vi "SetFrameTime.vi"(3 "错误输入":errorcluster, 4 "IMAQdx Session In":T1, 5 "帧间隔/us":i64) -> (0 "错误输出":errorcluster, 1 "IMAQdx Session Out":T1, 2 "帧率/FPS":dbl)   [LabVIEW 2012]
uses:
  <vilib>/userDefined/High Color/IMAQdx.ctl
  <resource>/objmgr/imaqdx.rc
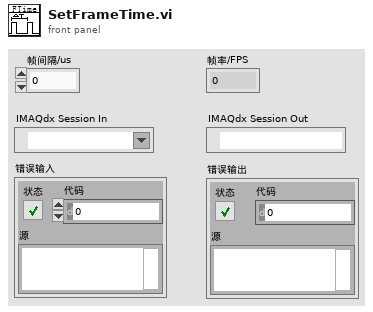
[diagram p1: front panel]
types:
  T1 = typedef "IMAQdx.ctl" = refnum<k21>
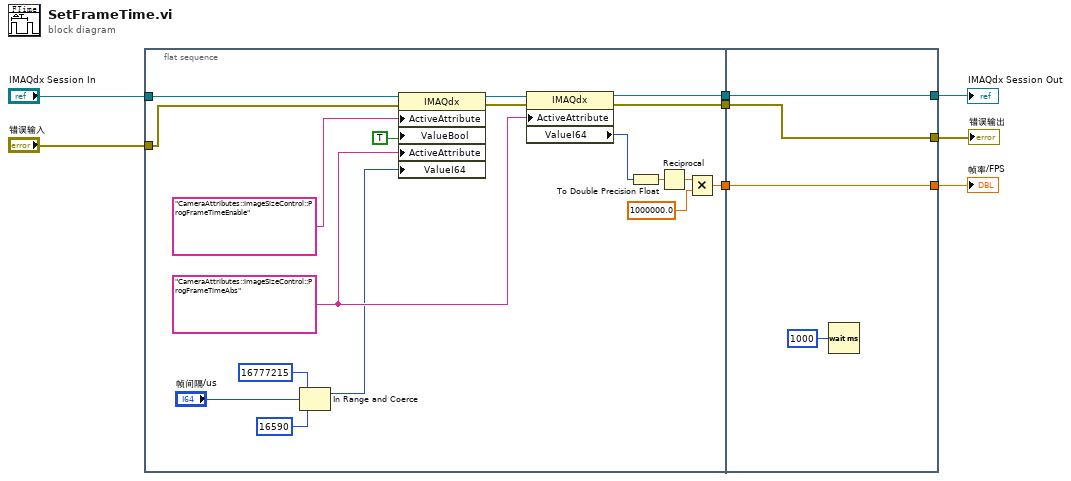
[diagram p0: block diagram]
diagram:
  n1 = flat-sequence {
    tunnel: "IMAQdx Session In" -> [w13]
    tunnel: "错误输入" -> [w12]
    tunnel: [w11] -> w6
    tunnel: [w10] -> w4
    tunnel: [w9] -> w2
    tunnel: [w29] -> w5
    tunnel: w6 -> [w29]
    tunnel: [w28] -> w3
    tunnel: w4 -> [w28]
    tunnel: w2 -> [w27]
    tunnel: [w27] -> w1
    frame #0 {
      w22 = "CameraAttributes::ImageSizeControl::ProgFrameTimeAbs" ("ActiveAttribute")
      n2 = In Range and Coerce(upper limit=i64 16777215 ("下限"), x="帧间隔/us", lower limit=i64 16590 ("上限")) -> (coerced(x)=w21:i64)  [unwired: 1 out]
      n3 = property class="IMAQdx"(reference=w13, error in=w12, "ActiveAttribute"="CameraAttributes::ImageSizeControl::ProgFrameTimeEnable", "ValueBool"=TRUE, "ActiveAttribute"=w22, "ValueI64"=w21) -> (reference out=w16:T1, error out=w17:errorcluster)
      n4 = property class="IMAQdx"(reference=w16, error in=w17, "ActiveAttribute"=w22) -> (reference out=w9:T1, error out=w10:errorcluster, "ValueI64"=w24:i64)
      n5 = To Double Precision Float(number=w24) -> (double precision float=w23:dbl)
      n6 = Reciprocal(x=w23) -> (1/x=w25:dbl)
      n7 = Multiply(x=w25, y=1000000.0) -> (x*y=w11:dbl)
    }
    frame #1 {
      n8 = Wait (ms)(milliseconds to wait=u32 1000 ("等待时间（毫秒）")) -> ()  [unwired: 1 out]
    }
  }
  "IMAQdx Session Out" <- w1
  "错误输出" <- w3
  "帧率/FPS" <- w5
